vi "ConvertRefToProtocolType.vi"(11 "Array (Eingang)":refnum<vi>) -> (0 "Fehler (Ausgang)":errorcluster, 2 "ProtocolT":T1 {"Zeitstempel" format=" %<%X %x>T"}, 3 "Array (Ausgang)":refnum<vi>)   [LabVIEW 2014]
uses:
  controls/ProtocolT.ctl
  controls/ProtocolEntry.ctl
panel:
  in  "Fehler Eingang":errorcluster caption="Fehler (Eingang, kein Fehler)"
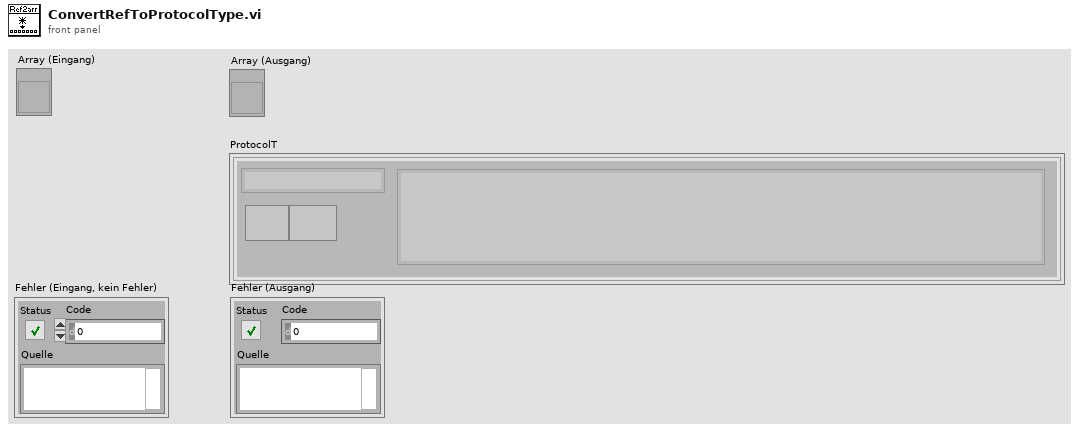
[diagram p1: front panel]
types:
  T1 = typedef "ProtocolT.ctl" = T2[]
  T2 = typedef "ProtocolEntry.ctl" = cluster{"Zeitstempel":timestamp, "String":string, "Abbrechen-Schaltfläche":bool, "Optionen-Schaltfläche":bool}
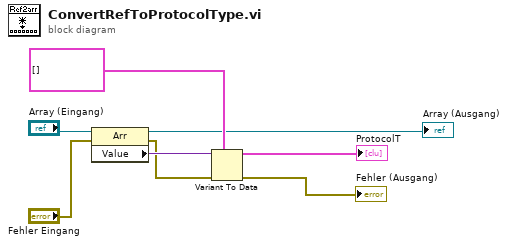
[diagram p0: block diagram]
diagram:
  n1 = property on="Eigenschaftsknoten" class="Arr"(reference="Array (Eingang)", error in="Fehler Eingang") -> (reference out=→"Array (Ausgang)":refnum<vi>, error out=w2:errorcluster, "Value"=w6:variant)
  n2 = Variant To Data(error in=w2, type=T1 [] ("ProtocolT"), Variant=w6) -> (data=→"ProtocolT":T1, error out=→"Fehler (Ausgang)":errorcluster)
